vi "get_ylims.vi"(6 "pad":dbl=0.25 format="%#_13g", 11 "amplitudes":dbl[](array[numeric])) -> (3 "ylims":dbl[](array[numeric]))   [LabVIEW 2017]
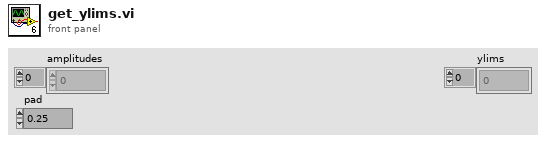
[diagram p1: front panel]
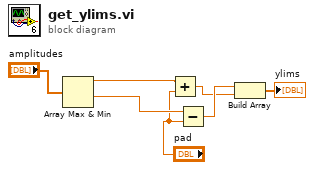
[diagram p0: block diagram]
diagram:
  n1 = Array Max & Min(array="amplitudes") -> (max value=w5:dbl, min value=w4:dbl)  [unwired: 2 out]
  n2 = Add(x=w5, y="pad") -> (x+y=w6:dbl)
  n3 = Subtract(x=w4, y="pad") -> (x-y=w7:dbl)
  n4 = Build Array(w7, w6) -> (→"ylims":dbl[])
